vi "PromptWithMessage.vi"(0 "Enable":bool=TRUE, 2 "String":string="Prompt Here", 5 "error in (no error)":errorcluster) -> (17 "Index":dbl format="%#g", 18 "OK":bool, 19 "error out":errorcluster)   [LabVIEW 2018]
doc: "Displays a standard dialog box that prompts users to enter information, such as a user name and password.\n--------------------\n\nThis Express VI is configured as follows:\n\nMessage to Display to the User:Prompt Here\nThe inputs are: \nNumber: Index"
panel:
  in  "Index":dbl format="%#g"
  in  "Cancel":bool
  in  "OK2":bool
  in  "OK1":bool
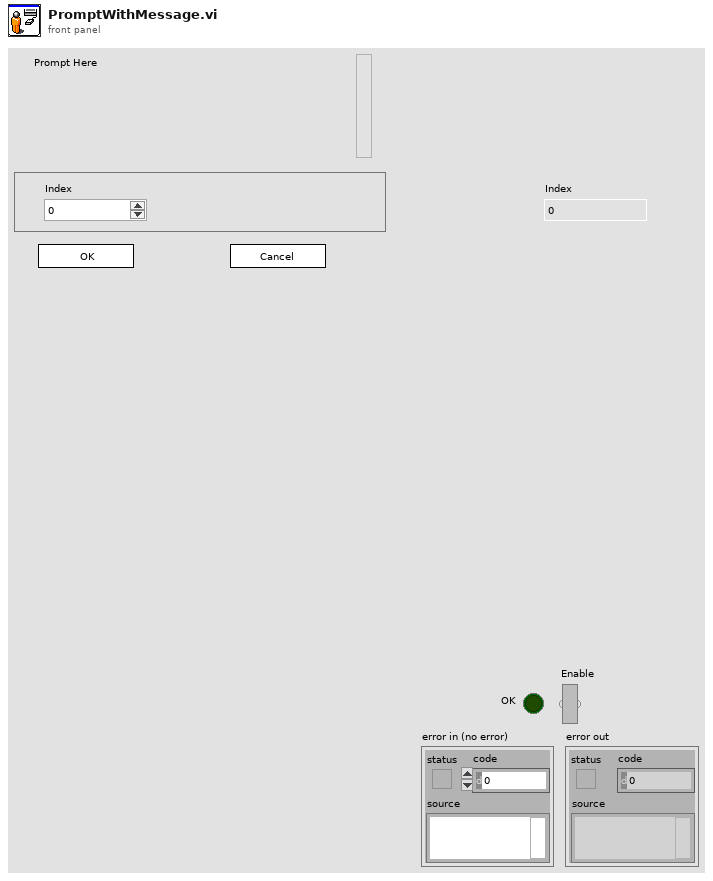
[diagram p1: front panel]
types:
  T1 = cluster{"Input Name":string, "Input Data Type":i32}[]
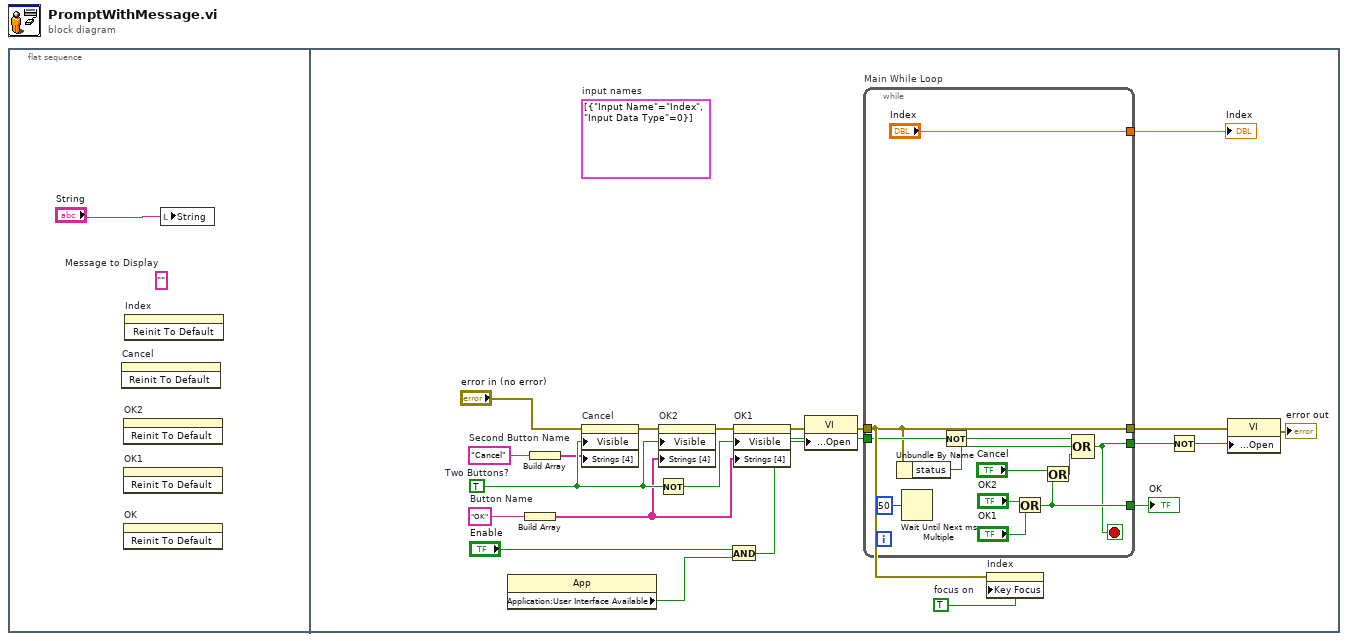
[diagram p0: block diagram]
diagram:
  n1 = flat-sequence {
    frame #0 {
      (unwired) ""  # Message to Display
      n2 = invoke on="Cancel" class="Bool" method="Reinit To Default"() -> ()  [unwired: 3 in, 3 out]
      n3 = invoke on="OK2" class="Bool" method="Reinit To Default"() -> ()  [unwired: 3 in, 3 out]
      n4 = invoke on="OK1" class="Bool" method="Reinit To Default"() -> ()  [unwired: 3 in, 3 out]
      n5 = invoke on="OK" class="Bool (strict)" method="Reinit To Default"() -> ()  [unwired: 3 in, 3 out]
      n6 = invoke on="Index" class="DigNum (strict)" method="Reinit To Default"() -> ()  [unwired: 3 in, 3 out]
      n7 = local write "String"("String") -> ()
    }
    frame #1 {
      w3 = TRUE  # focus on
      (unwired) T1 [{"Input Name"="Index", "Input Data Type"=0}]  # input names
      w15 = "Cancel"  # Second Button Name
      w13 = "OK"  # Button Name
      w22 = TRUE  # Two Buttons?
      n8 = property class="App"() -> ("Application:User Interface Available"=w5:bool)  [unwired: 2 in, 2 out]
      n9 = Build Array(w13) -> (w14:string[])
      n10 = Build Array(w15) -> (w16:string[])
      n11 = property on="Cancel" class="Bool"(error in="error in (no error)", "Visible"=w22, "Strings [4]"=w16) -> (error out=w19:errorcluster)  [unwired: 1 in, 1 out]
      n12 = Not(x=w22) -> (.not. x?=w20:bool)
      n13 = property on="OK2" class="Bool"(error in=w19, "Visible"=w22, "Strings [4]"=w14) -> (error out=w18:errorcluster)  [unwired: 1 in, 1 out]
      n14 = And(x="Enable", y=w5) -> (x .and. y?=w6:bool)
      n15 = property on="OK1" class="Bool"(error in=w18, "Visible"=w20, "Strings [4]"=w14) -> (error out=w12:errorcluster)  [unwired: 1 in, 1 out]
      n16 = property class="VI"(error in=w12, "Front Panel Window:Open"=w6) -> (error out=w11:errorcluster)  [unwired: 1 in, 1 out]
      n17 = while "Main While Loop" {
        tunnel: [w31] -> w21
        tunnel: w6 -> [w29]
        tunnel: [w27] -> w17
        tunnel: w11 -> [w26]
        tunnel: [w26] -> w9
        tunnel: ["Index"] -> w4
        stop <- w27 stop-if-true
        n18 = Unbundle By Name(w26) -> ("status"=w24:bool)
        n19 = Wait Until Next ms Multiple(millisecond multiple=u32 50) -> ()  [unwired: 1 out]
        n20 = Not(x=w29) -> (.not. x?=w28:bool)
        n21 = Or(x="OK2", y="OK1") -> (x .or. y?=w31:bool)
        n22 = Or(x="Cancel", y=w31) -> (x .or. y?=w25:bool)
        n23 = Compound Arithmetic op=OR(w28, w24, w25) -> (w27:bool)
      }
      "OK" <- w21
      "Index" <- w4
      n24 = property on="Index" class="DigNum (strict)"(error in=w11, "Key Focus"=w3) -> ()  [unwired: 1 in, 2 out]
      n25 = Not(x=w17) -> (.not. x?=w2:bool)
      n26 = property class="VI"(error in=w9, "Front Panel Window:Open"=w2) -> (error out=→"error out":errorcluster)  [unwired: 1 in, 1 out]
    }
  }
